vi "PhysName2AxisNo.vi"(8 "error in (no error)":errorcluster, 10 "PhysicalChannelName":string, 11 "CS++Motor in":refnum<class "CS++Motor.lvclass">) -> (0 "error out":errorcluster, 2 "AxisNumber":u8, 3 "CS++Motor out":refnum<class "CS++Motor.lvclass">)   [LabVIEW 2015, in "CS++Motor.lvlib" / "CS++Motor.lvclass"]
doc: "This small utility VI needs the physical Name of the channel and returns the axis number (0...N-1). Sometimes this is needed in a child class of CS++Motor.lvclass."
uses:
  CS++Motor.lvclass
  CS++Motor.lvclass/CS++Motor.ctl
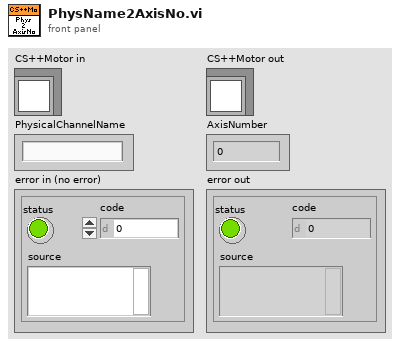
[diagram p1: front panel]
types:
  T1 = cluster{"LogicalName":string, "PhysicalName":string, "unit":string, "Scaling":dbl, "StartVelocity":dbl, "StopVelocity":dbl, "Acceleration":dbl, "RangeMin":dbl, "RangeMax":dbl, "LogicalPos-Array":cluster{"LogicalPosition":string, "SetPosition":dbl}[]}[]
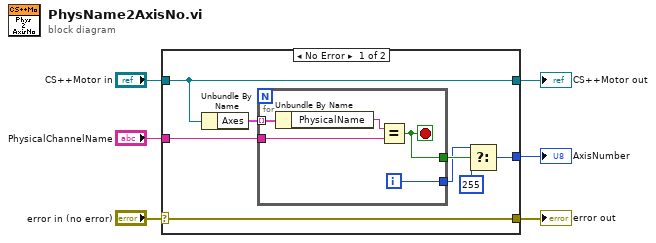
[diagram p0: block diagram]
diagram:
  n1 = case shown="No Error" "error in (no error)" {
    selector: "error in (no error)" -> [w14 w21]
    tunnel: [w14 w21] -> w5
    tunnel: [w13 w20] -> w3
    tunnel: "CS++Motor in" -> [w13 w20]
    tunnel: "PhysicalChannelName" -> [w11 _]
    tunnel: [w8 _] -> w1
    frame No Error {
      n2 = Unbundle By Name(w13) -> ("Axes"=w12:T1)
      n3 = for {
        tunnel: w12 -> [w19] mode=indexing
        tunnel: w11 -> [w17]
        tunnel: [w16] -> w9
        tunnel: [w15] -> w10
        i -> [w16]
        stop <- w15 stop-if-true
        n4 = Unbundle By Name(w19) -> ("PhysicalName"=w18:string)
        n5 = Equal?(x=w18, y=w17) -> (x = y?=w15:bool)
      }
      n6 = Select(t=w9, s=w10, f=u8 255 ("AxisNumber")) -> (s? t:f=w8:i32)
    }
    frame Error {
    }
  }
  "error out" <- w5
  "CS++Motor out" <- w3
  "AxisNumber" <- w1
